vi "ObtenerFilaEnUso.vi"(10 "Tabla in":string[][](array[string]), 11 "Frecuencia":string) -> (3 "index of element":i32)   [LabVIEW 2019, in "Prueba33.lvclass"]
uses:
  Prueba33.lvclass
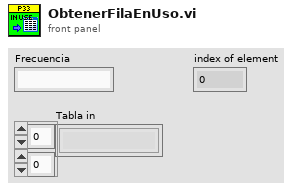
[diagram p1: front panel]
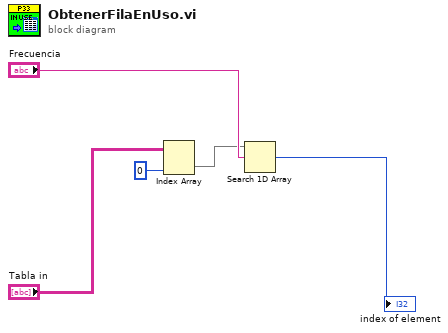
[diagram p0: block diagram]
diagram:
  n1 = Index Array(array="Tabla in", index (col)=0 ("disabled index (col)")) -> (element=w2:string[])  [unwired: 1 in]
  n2 = Search 1D Array(1D array=w2, element="Frecuencia") -> (index of element=→"index of element":i32)  [unwired: 1 in]
